vi "EncAlg - addon.vi"(10 "EnValIn":dbl[](array[numeric]), 11 "element":T1) -> (0 "VelValOut":dbl[](array[numeric]), 1 "0, 1":i16, 2 "logical AND":bool)   [LabVIEW 2019]
panel:
  out "appended mere":dbl[](array[numeric])
  out "Sense":dbl
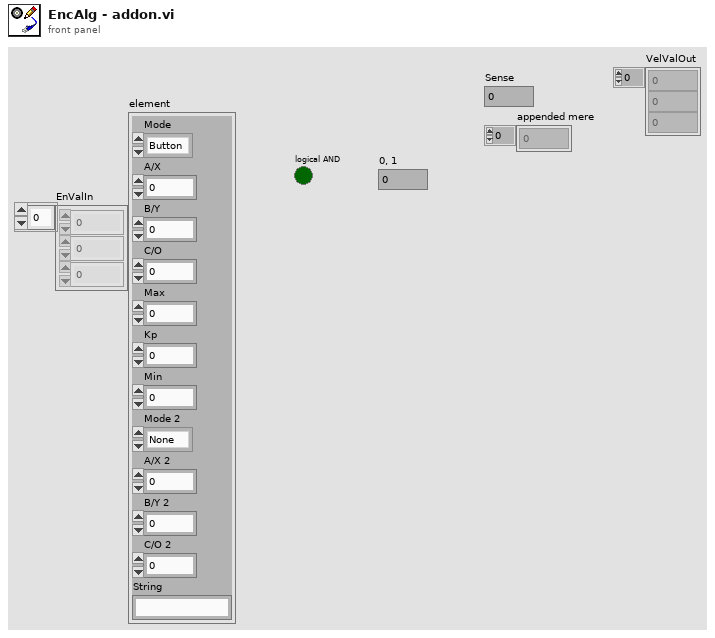
[diagram p1: front panel]
types:
  T1 = cluster{"Mode":enum16{"Button", "Encoder", "Delay", "IR Stop", "Line Stop"}, "A/X":dbl, "B/Y":dbl, "C/O":dbl, "Max":dbl, "Kp":dbl, "Min":dbl, "Mode 2":enum16{"None", "IR Stabilize", "Line Stabilize", "Encoder", "IR Stop", "Servo"}, "A/X 2":dbl, "B/Y 2":dbl, "C/O 2":dbl, "String":string}
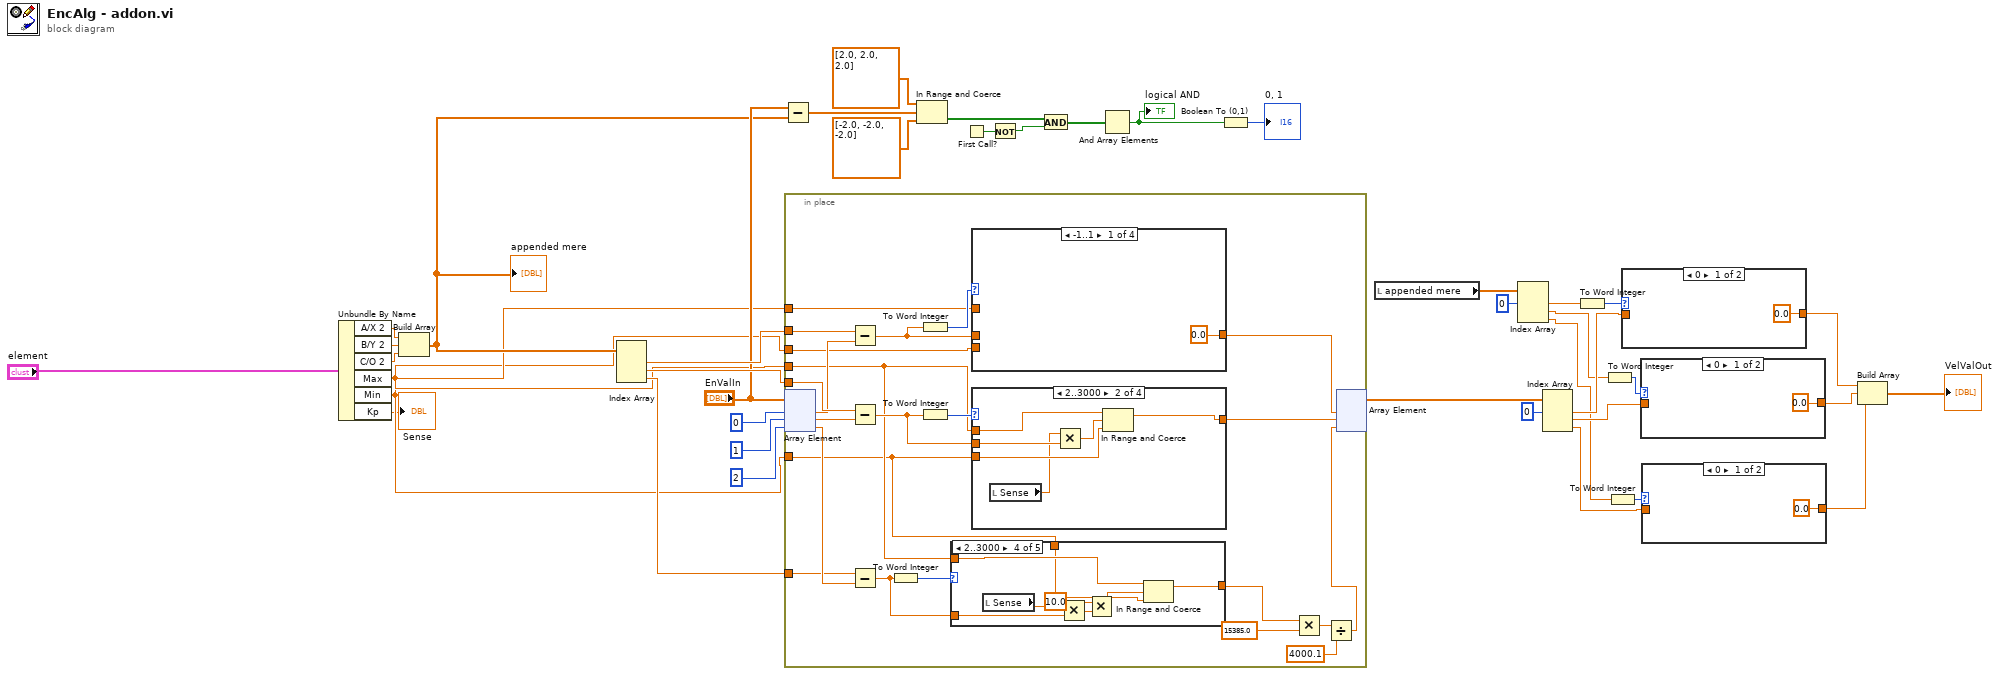
[diagram p0: block diagram]
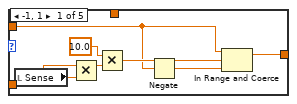
[diagram p5: hidden frame]
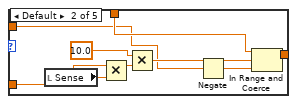
[diagram p6: hidden frame]
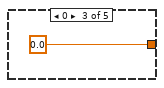
[diagram p7: hidden frame]
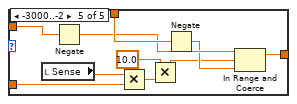
[diagram p8: hidden frame]
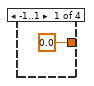
[diagram p9: hidden frame]
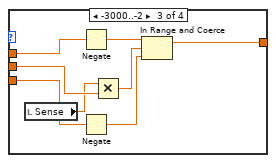
[diagram p10: hidden frame]
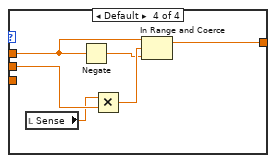
[diagram p11: hidden frame]
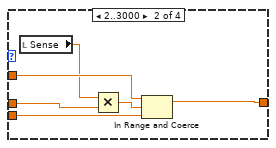
[diagram p12: hidden frame]
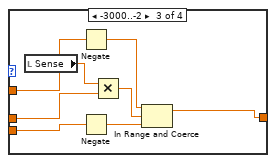
[diagram p13: hidden frame]
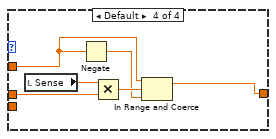
[diagram p14: hidden frame]
diagram:
  n1 = Unbundle By Name("element") -> ("A/X 2"=w24:dbl, "B/Y 2"=w23:dbl, "C/O 2"=w22:dbl, "Max"=w21:dbl, "Min"=w20:dbl, "Kp"=→"Sense":dbl)
  n2 = Build Array(w24, w23, w22) -> (w25:dbl[])
  "appended mere" <- w25
  n3 = Index Array(array=w25) -> (element #1=w37:dbl, element #2=w41:dbl, element #3=w36:dbl)  [unwired: 3 in]
  n4 = Subtract(x="EnValIn", y=w25) -> (x-y=w35:dbl[])
  n5 = in-place {
    in-place-border: w41 -> [w63]
    in-place-border: w37 -> [w61]
    in-place-border: w36 -> [w59]
    in-place-border: w21 -> [w53]
    in-place-border: w20 -> [w52]
    in-place-border: w21 -> [w49]
    in-place-border: w20 -> [w48]
    n6 = in-place-array #1("EnValIn", 0, 1, 2) -> (w62:dbl, w64:dbl, w60:dbl)
    n7 = Subtract(x=w61, y=w62) -> (x-y=w51:dbl)
    n8 = Subtract(x=w63, y=w64) -> (x-y=w50:dbl)
    n9 = Subtract(x=w59, y=w60) -> (x-y=w47:dbl)
    n10 = To Word Integer(number=w47) -> (16bit integer=w56:i16)
    n11 = To Word Integer(number=w51) -> (16bit integer=w54:i16)
    n12 = To Word Integer(number=w50) -> (16bit integer=w55:i16)
    n13 = case shown="2..3000" w56 {
      tunnel: w47 -> [w69 w78 _ w88 w98]
      tunnel: [w70 w79 0.0 ("x") w89 w99] -> w43
      tunnel: w49 -> [w66 w74 _ w86 w96]
      tunnel: w48 -> [_ w75 _ w85 w95]
      frame -1, 1 {
        n14 = local read "Sense"() -> (w67:dbl)
        n15 = Multiply(x=w69, y=w67) -> (x*y=w68:dbl)
        n16 = Multiply(x=10.0, y=w68) -> (x*y=w72:dbl)
        n17 = Negate(x=w66) -> (-x=w65:dbl)
        n18 = In Range and Coerce(upper limit=w66, x=w72, lower limit=w65) -> (coerced(x)=w70:dbl)  [unwired: 1 out]
      }
      frame Default {
        n19 = local read "Sense"() -> (w76:dbl)
        n20 = Multiply(x=w78, y=w76) -> (x*y=w77:dbl)
        n21 = Multiply(x=10.0, y=w77) -> (x*y=w81:dbl)
        n22 = Negate(x=w74) -> (-x=w73:dbl)
        n23 = In Range and Coerce(upper limit=w75, x=w81, lower limit=w73) -> (coerced(x)=w79:dbl)  [unwired: 1 out]
      }
      frame 0 {
      }
      frame 2..3000 {
        n24 = local read "Sense"() -> (w87:dbl)
        n25 = Multiply(x=w87, y=w88) -> (x*y=w90:dbl)
        n26 = Multiply(x=10.0, y=w90) -> (x*y=w84:dbl)
        n27 = In Range and Coerce(upper limit=w86, x=w84, lower limit=w85) -> (coerced(x)=w89:dbl)  [unwired: 1 out]
      }
      frame -3000..-2 {
        n28 = local read "Sense"() -> (w97:dbl)
        n29 = Negate(x=w96) -> (-x=w94:dbl)
        n30 = Multiply(x=w97, y=w98) -> (x*y=w100:dbl)
        n31 = Multiply(x=10.0, y=w100) -> (x*y=w92:dbl)
        n32 = Negate(x=w95) -> (-x=w93:dbl)
        n33 = In Range and Coerce(upper limit=w94, x=w92, lower limit=w93) -> (coerced(x)=w99:dbl)  [unwired: 1 out]
      }
    }
    n34 = case shown="-1..1" w54 {
      tunnel: w51 -> [_ w126 w134 w140]
      tunnel: [0.0 ("x") w127 w135 w141] -> w58
      tunnel: w53 -> [_ w125 w133 w139]
      tunnel: w52 -> [_ w124 w131 _]
      frame -1..1 {
      }
      frame 2..3000 {
        n35 = local read "Sense"() -> (w123:dbl)
        n36 = Multiply(x=w123, y=w126) -> (x*y=w128:dbl)
        n37 = In Range and Coerce(upper limit=w125, x=w128, lower limit=w124) -> (coerced(x)=w127:dbl)  [unwired: 1 out]
      }
      frame -3000..-2 {
        n38 = local read "Sense"() -> (w129:dbl)
        n39 = Negate(x=w133) -> (-x=w130:dbl)
        n40 = Negate(x=w131) -> (-x=w132:dbl)
        n41 = Multiply(x=w129, y=w134) -> (x*y=w136:dbl)
        n42 = In Range and Coerce(upper limit=w130, x=w136, lower limit=w132) -> (coerced(x)=w135:dbl)  [unwired: 1 out]
      }
      frame Default {
        n43 = local read "Sense"() -> (w137:dbl)
        n44 = Negate(x=w139) -> (-x=w138:dbl)
        n45 = Multiply(x=w137, y=w140) -> (x*y=w142:dbl)
        n46 = In Range and Coerce(upper limit=w139, x=w142, lower limit=w138) -> (coerced(x)=w141:dbl)  [unwired: 1 out]
      }
    }
    n47 = case shown="2..3000" w55 {
      tunnel: w50 -> [_ w105 w113 w119]
      tunnel: [0.0 ("x") w106 w114 w120] -> w57
      tunnel: w49 -> [_ w104 w109 w117]
      tunnel: w48 -> [_ w103 w110 _]
      frame -1..1 {
      }
      frame 2..3000 {
        n48 = local read "Sense"() -> (w102:dbl)
        n49 = Multiply(x=w102, y=w105) -> (x*y=w107:dbl)
        n50 = In Range and Coerce(upper limit=w104, x=w107, lower limit=w103) -> (coerced(x)=w106:dbl)  [unwired: 1 out]
      }
      frame -3000..-2 {
        n51 = local read "Sense"() -> (w108:dbl)
        n52 = Negate(x=w109) -> (-x=w112:dbl)
        n53 = Negate(x=w110) -> (-x=w111:dbl)
        n54 = Multiply(x=w108, y=w113) -> (x*y=w115:dbl)
        n55 = In Range and Coerce(upper limit=w112, x=w115, lower limit=w111) -> (coerced(x)=w114:dbl)  [unwired: 1 out]
      }
      frame Default {
        n56 = local read "Sense"() -> (w116:dbl)
        n57 = Negate(x=w117) -> (-x=w118:dbl)
        n58 = Multiply(x=w116, y=w119) -> (x*y=w121:dbl)
        n59 = In Range and Coerce(upper limit=w117, x=w121, lower limit=w118) -> (coerced(x)=w120:dbl)  [unwired: 1 out]
      }
    }
    n60 = Multiply(x=w43, y=15385.0) -> (x*y=w46:dbl)
    n61 = Divide(x=w46, y=4000.1) -> (x/y=w42:dbl)
    n62 = in-place-array #1(w58, w57, w42) -> (w16:dbl[])  [unwired: 3 out]
  }
  n63 = In Range and Coerce(upper limit=dbl[] [2.0, 2.0, 2.0], x=w35, lower limit=dbl[] [-2.0, -2.0, -2.0]) -> (In Range?=w32:bool[])  [unwired: 1 out]
  n64 = First Call?() -> (First Call?: T/F=w31:bool)
  n65 = Not(x=w31) -> (.not. x?=w30:bool)
  n66 = And(x=w32, y=w30) -> (x .and. y?=w29:bool[])
  n67 = And Array Elements(Boolean array=w29) -> (logical AND=w28:bool)
  "logical AND" <- w28
  n68 = Boolean To (0,1)(Boolean=w28) -> (0, 1=→"0, 1":i16)
  n69 = local read "appended mere"() -> (w18:dbl[])
  n70 = Index Array(array=w18, index #1=0 ("index")) -> (element #1=w8:dbl, element #2=w7:dbl, element #3=w4:dbl)  [unwired: 2 in]
  n71 = Index Array(array=w16, index #1=0 ("index")) -> (element #1=w9:dbl, element #2=w6:dbl, element #3=w5:dbl)  [unwired: 2 in]
  n72 = To Word Integer(number=w8) -> (16bit integer=w14:i16)
  n73 = To Word Integer(number=w7) -> (16bit integer=w12:i16)
  n74 = To Word Integer(number=w4) -> (16bit integer=w10:i16)
  n75 = case shown="0" w14 {
    tunnel: [0.0 w144] -> w13
    tunnel: w9 -> [_ w144]
    frame 0 {
    }
    frame Default {
    }
  }
  n76 = case shown="0" w12 {
    tunnel: [0.0 w146] -> w11
    tunnel: w6 -> [_ w146]
    frame 0 {
    }
    frame Default {
    }
  }
  n77 = case shown="0" w10 {
    tunnel: [0.0 w148] -> w3
    tunnel: w5 -> [_ w148]
    frame 0 {
    }
    frame Default {
    }
  }
  n78 = Build Array(w13, w11, w3) -> (→"VelValOut":dbl[])
